vi "RichToFlatcif_manager_DestroyPluginLoaderRequest.vi"(5 "OutputClusterType":T1, 11 "InputCluster":T2) -> (3 "OutputCluster":T1)   [LabVIEW 2021, in "CIF_Manager_client.lvlib"]
uses:
  CIF_Manager_client.lvlib
  cif_manager_DestroyPluginLoaderRequest.ctl
  cif_manager_DestroyPluginLoaderRequest_Flat.ctl
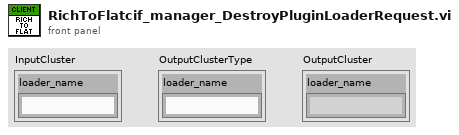
[diagram p1: front panel]
types:
  T1 = typedef "CIF_Manager_client.lvlib/cif_manager_DestroyPluginLoaderRequest_Flat.ctl" = cluster{"loader_name":string}
  T2 = typedef "CIF_Manager_client.lvlib/cif_manager_DestroyPluginLoaderRequest.ctl" = cluster{"loader_name":string}
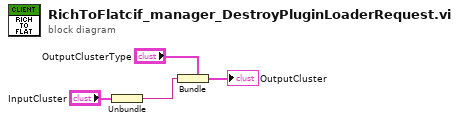
[diagram p0: block diagram]
diagram:
  n1 = Unbundle "Unbundle"("InputCluster") -> ("loader_name"=w1:string)
  n2 = Bundle "Bundle"(cluster="OutputClusterType", "loader_name"=w1) -> (→"OutputCluster":T1)
